vi "Verdi-V5-Main.vi"() -> ()   [LabVIEW 2019]
panel:
  in  "Laser":bool
  out "Power":string
  out "Shutter":bool
  out "Laser":bool
  out "StatusBar":string
  in  "Custom Command":string
  in  "Exit":bool
  in  "Resource":refnum<visa-resource-name>
  out "Response":string
  in  "Query":bool
  in  "Write":bool
  in  "Shutter":bool
  # "Verdi-V5 Control"
  # "W"
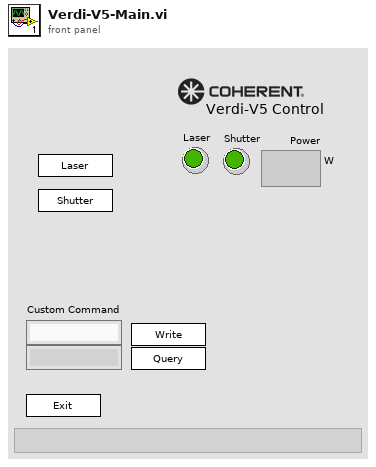
[diagram p1: front panel]
types:
  T1 = enum32{"Invalid", "Standard", "Closed", "Hidden", "Minimized", "Maximized"}
  T2 = enum32{"invalid app kind", "Development System", "Run Time System", "Student Edition", "Embedded LabVIEW", "Evaluation", "Custom"}
  T3 = cluster{"Core":cluster{"Current VI Reference":refnum<vi>, "Close Panel on Exit?":bool}, "Your Boolean data":bool, "Your string data":string, "Resource":refnum<visa-resource-name>}
  T4 = cluster{"Current VI Reference":refnum<vi>, "Close Panel on Exit?":bool}
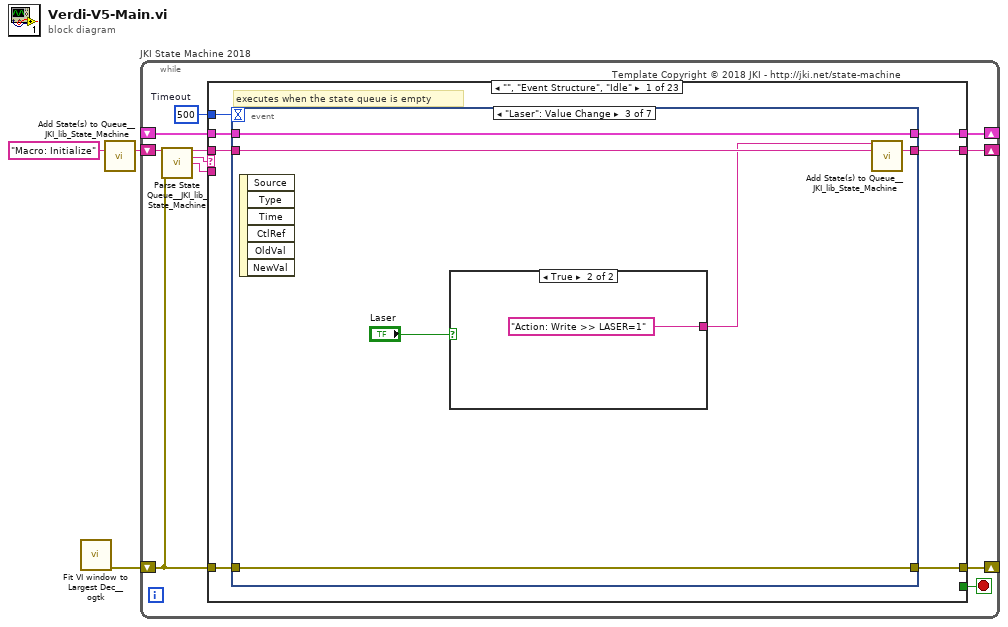
[diagram p0: block diagram]
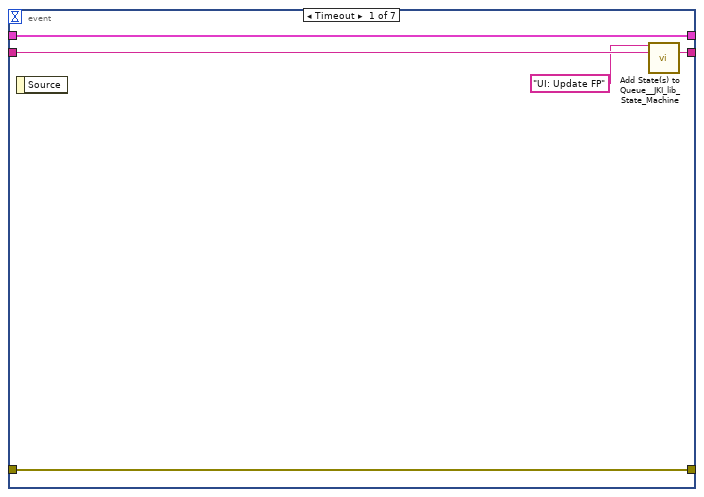
[diagram p2: hidden frame]
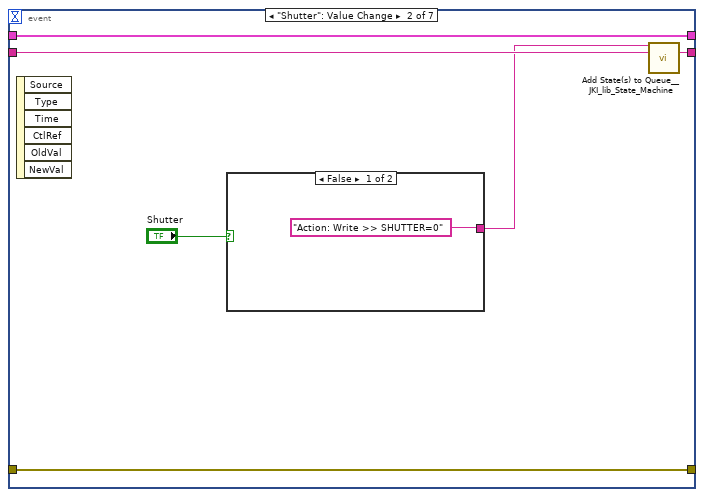
[diagram p3: hidden frame]
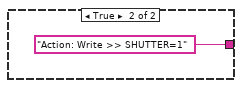
[diagram p4: hidden frame]
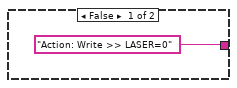
[diagram p5: hidden frame]
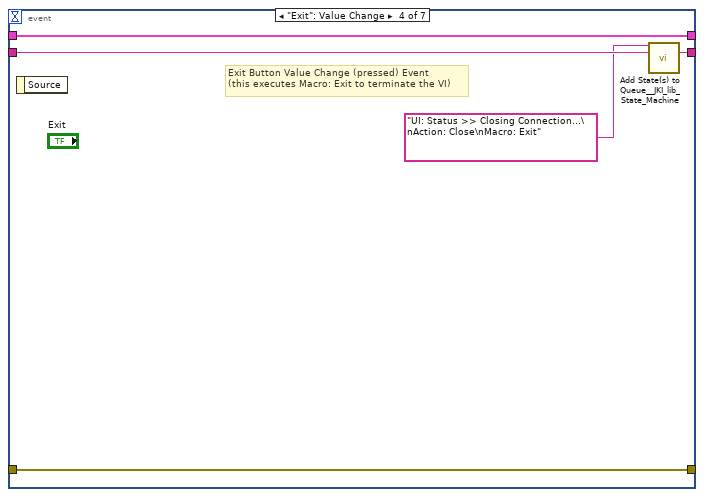
[diagram p6: hidden frame]
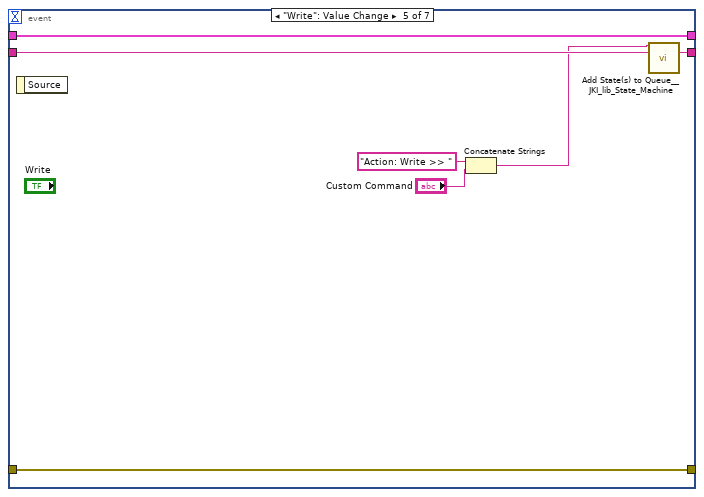
[diagram p7: hidden frame]
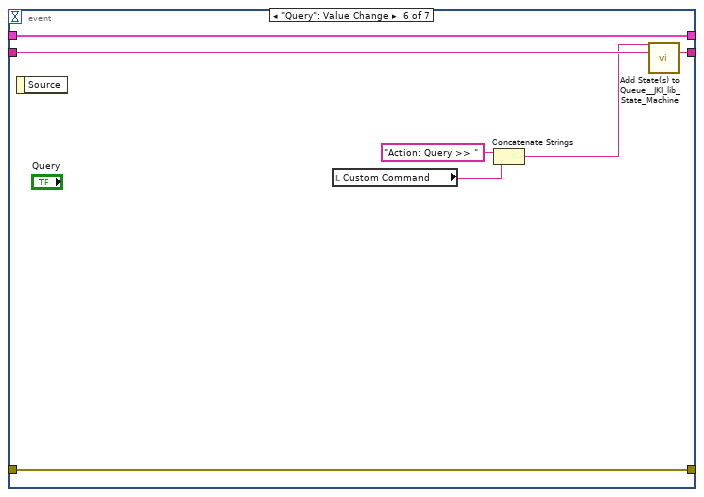
[diagram p8: hidden frame]
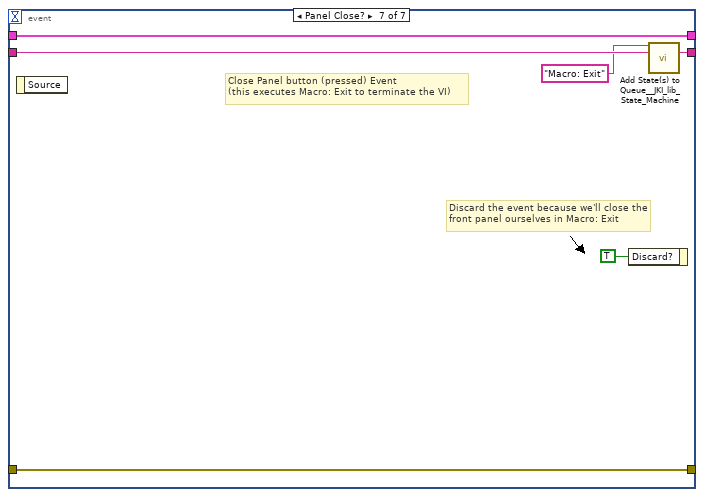
[diagram p9: hidden frame]
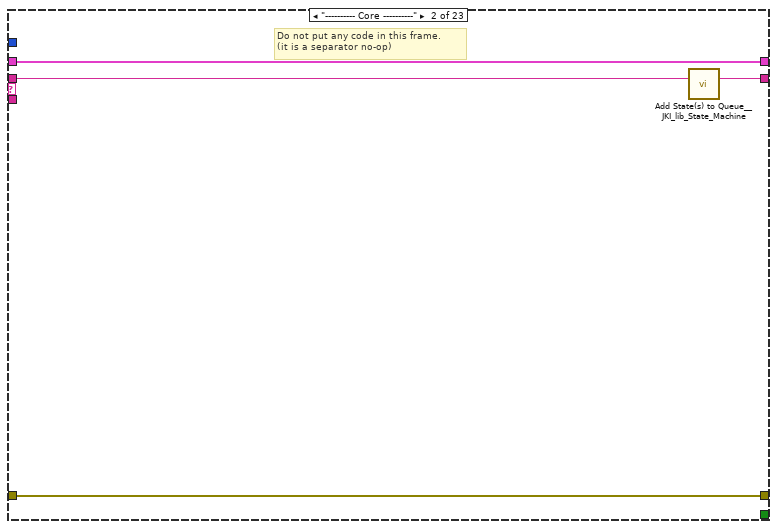
[diagram p10: hidden frame]
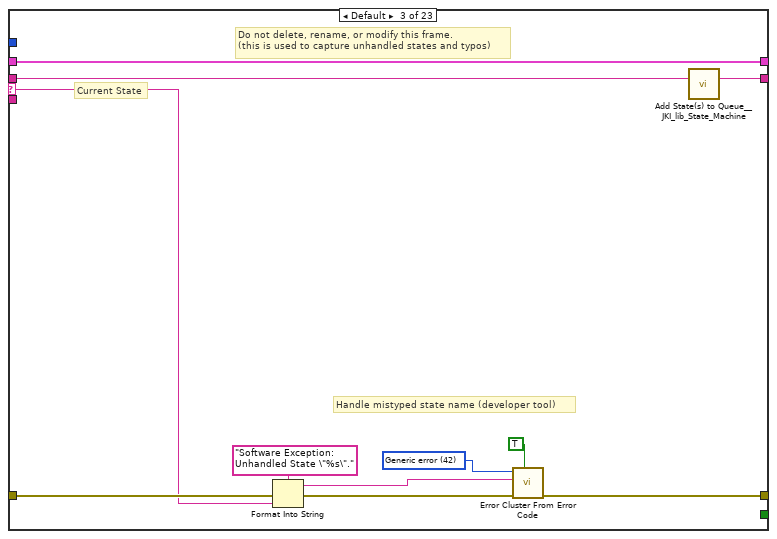
[diagram p11: hidden frame]
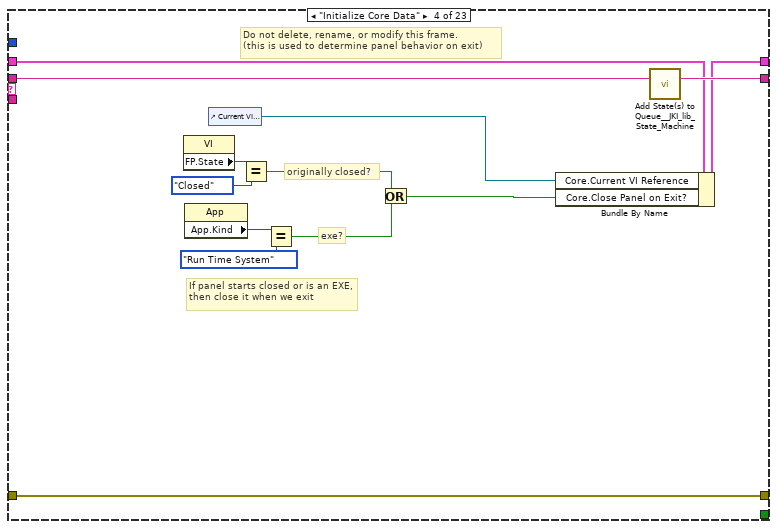
[diagram p12: hidden frame]
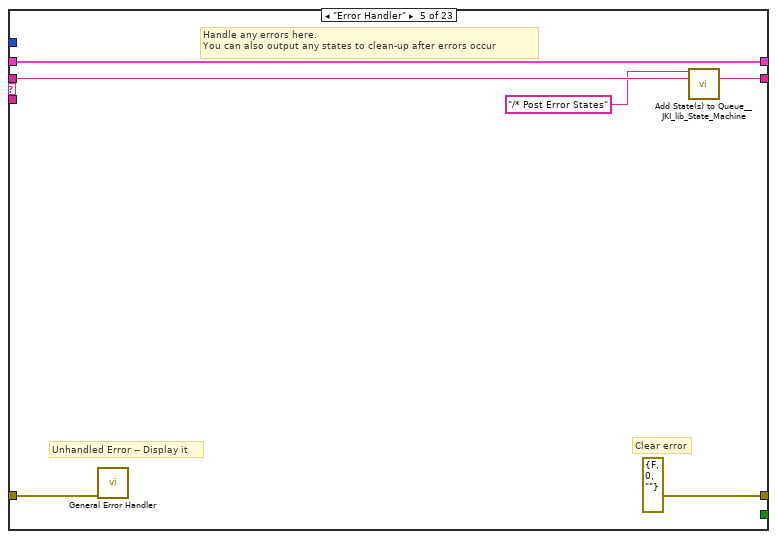
[diagram p13: hidden frame]
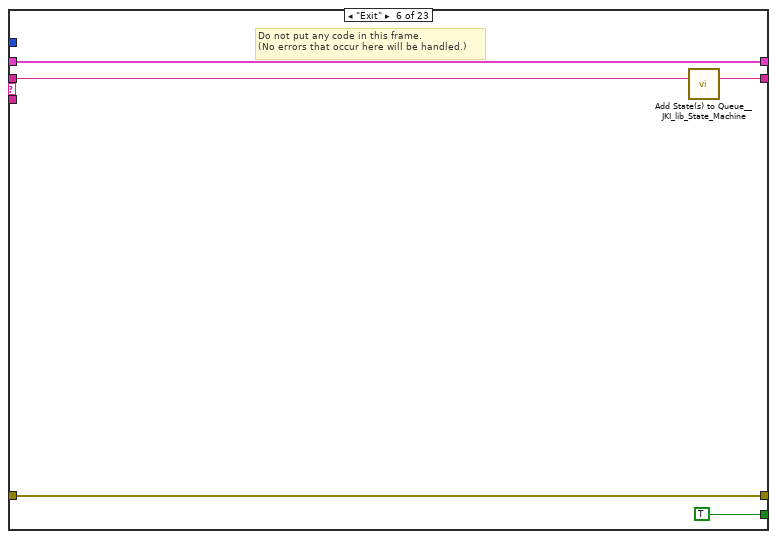
[diagram p14: hidden frame]
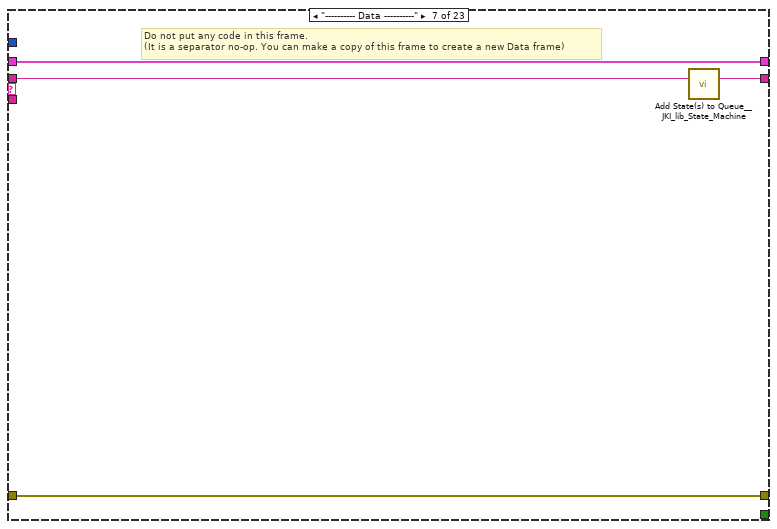
[diagram p15: hidden frame]
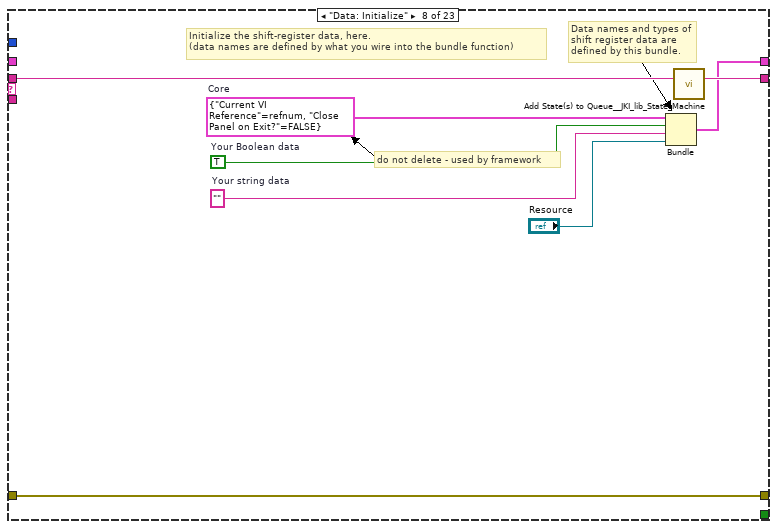
[diagram p16: hidden frame]
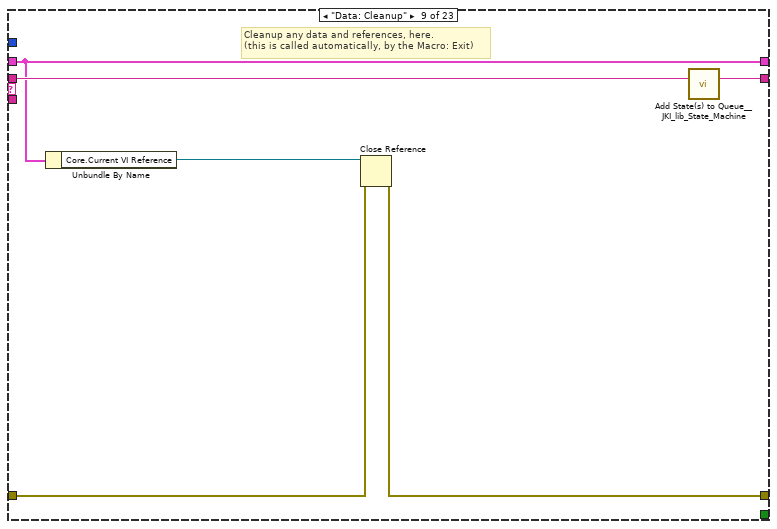
[diagram p17: hidden frame]
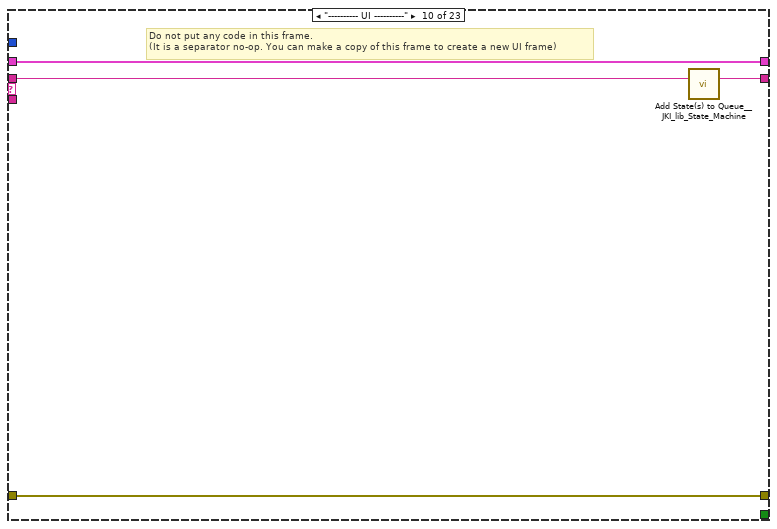
[diagram p18: hidden frame]
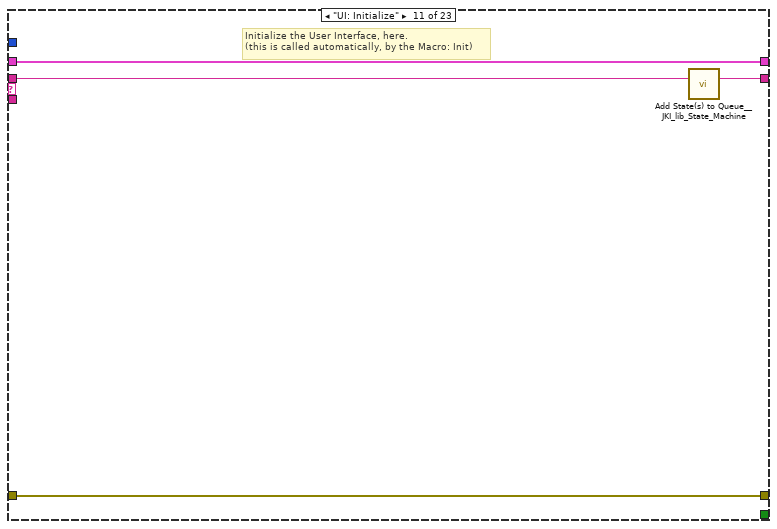
[diagram p19: hidden frame]
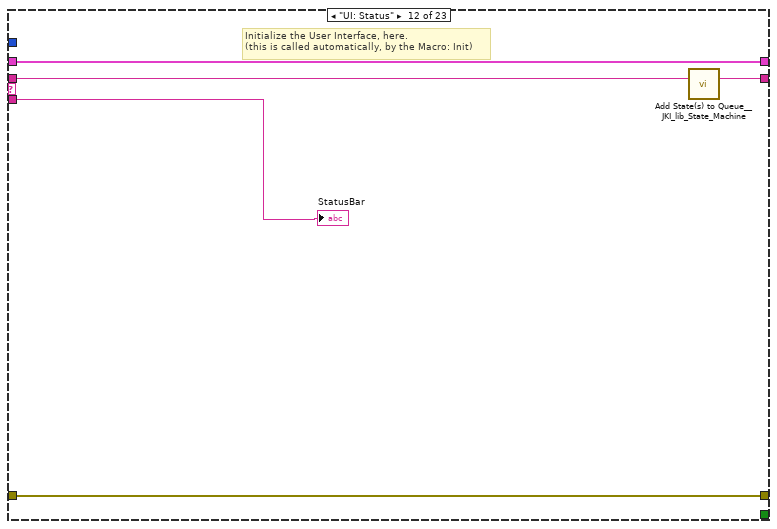
[diagram p20: hidden frame]
diagram:
  n1 = call <userlib>:"Fit VI window to Largest Dec__ogtk.vi"() -> ("error out"=w1:errorcluster)  [unwired: 6 in, 1 out]
  n2 = call <vilib>:"Add State(s) to Queue__JKI_lib_State_Machine.vi"("State(s) in (\"\")"="Macro: Initialize") -> ("States Out"=w3:string)  [unwired: 14 in]
  n3 = while "JKI State Machine 2018" {
    shift-right: [w7] -> _
    shift-left: _ -> [w6]
    shift-right: [w10] -> _
    shift-left: w1 -> [w4]
    shift-right: [w9] -> _
    shift-left: w3 -> [w11]
    stop <- w8 stop-if-true
    w5 = 500  # Timeout
    # "Template Copyright © 2018 JKI - http://jki.net/state-machine"
    n4 = call <vilib>:"Parse State Queue__JKI_lib_State_Machine.vi"("State Queue"=w11, "Error In (no error)"=w4) -> ("Remaining States"=w13:string, "Current State"=w14:string, "Arguments"=w12:string)  [unwired: 11 in]
    n5 = case shown="\"\", \"Event Structure\", \"Idle\"" w14 {
      selector: w14 -> [_ _ w72 _ _ _ _ _ _ _ _ _ _ _ _ _ _ _ _ _ _ _ _]
      tunnel: w13 -> [w21 w71 w76 w95 w101 w106 w110 w118 w124 w128 w132 w137 w159 w165 w176 w245 w250 w260 w264 w274 w280 w289 w299]
      tunnel: w12 -> [_ _ _ _ _ _ _ _ _ _ _ w133 _ w160 w170 _ _ _ _ _ _ w281 w291]
      tunnel: w6 -> [w19 w68 w74 w88 w98 w104 w107 _ w119 w125 w130 w135 w153 w163 w172 w242 w247 w257 w261 w272 w278 w287 w297]
      tunnel: [w18 w69 w78 w92 errorcluster {"status"=FALSE, "code"=0, "source"=""} ("error out") w103 w108 w115 w120 w126 w129 w134 w150 w161 w173 w243 w248 w258 w262 w269 w277 w282 w295] -> w10
      tunnel: w4 -> [w17 w69 w77 w92 w97 w103 w108 w115 w121 w126 w129 w134 w157 w162 w174 w243 w248 w258 w262 w270 w276 w283 w294]
      tunnel: [w20 w70 w75 w94 w100 w105 w109 w117 w123 w127 w131 w136 w158 w164 w175 w244 w249 w259 w263 w273 w279 w288 w298] -> w9
      tunnel: [_ _ _ _ _ TRUE _ _ _ _ _ _ _ _ _ _ _ _ _ _ _ _ _] -> w8
      tunnel: [w16 w68 w74 w93 w98 w104 w107 w116 w119 w125 w130 w135 w152 w163 w172 w242 w247 w257 w261 w271 w278 w286 w296] -> w7
      tunnel: w5 -> [w15 _ _ _ _ _ _ _ _ _ _ _ _ _ _ _ _ _ _ _ _ _ _]
      frame "", "Event Structure", "Idle" {
        # "executes when the state queue is empty"
        n6 = event shown="[2] \"Laser\": Value Change" {
          selector: _ -> [_ _ _ _ _ _ _]
          dyn-events: _ -> [_ _ _ _ _ _ _]
          timeout: w15 -> [_ _ _ _ _ _ _]
          tunnel: w21 -> [w26 w32 w40 w47 w54 w61 w67]
          tunnel: [w25 w31 w39 w46 w53 w60 w66] -> w20
          tunnel: w19 -> [w23 w29 w37 w44 w51 w58 w64]
          tunnel: [w24 w30 w38 w45 w52 w59 w65] -> w18
          tunnel: w17 -> [w24 w30 w38 w45 w52 w59 w65]
          tunnel: [w23 w29 w37 w44 w51 w58 w64] -> w16
          event Timeout {
            n7 = event-data() -> ()  [unwired: 1 in, 1 out]
            n8 = call <vilib>:"Add State(s) to Queue__JKI_lib_State_Machine.vi"("State(s) in Front (\"\")"="UI: Update FP" ("State(s) in Front (\"\")"), "State(s) in (\"\")"=w26) -> ("States Out"=w25:string)  [unwired: 13 in]
          }
          event "Shutter": Value Change {
            n9 = event-data() -> ()  [unwired: 1 in, 6 out]
            n10 = case shown="False" "Shutter" {
              tunnel: ["Action: Write >> SHUTTER=0" "Action: Write >> SHUTTER=1"] -> w28
              frame False {
              }
              frame True {
              }
            }
            n11 = call <vilib>:"Add State(s) to Queue__JKI_lib_State_Machine.vi"("State(s) in Front (\"\")"=w28, "State(s) in (\"\")"=w32) -> ("States Out"=w31:string)  [unwired: 13 in]
          }
          event "Laser": Value Change {
            n12 = event-data() -> ()  [unwired: 1 in, 6 out]
            n13 = case shown="True" "Laser" {
              tunnel: ["Action: Write >> LASER=0" "Action: Write >> LASER=1"] -> w36
              frame False {
              }
              frame True {
              }
            }
            n14 = call <vilib>:"Add State(s) to Queue__JKI_lib_State_Machine.vi"("State(s) in Front (\"\")"=w36, "State(s) in (\"\")"=w40) -> ("States Out"=w39:string)  [unwired: 13 in]
          }
          event "Exit": Value Change {
            # "Exit Button Value Change (pressed) Event\n(this executes Macro: Exit to terminate the VI)"
            n15 = event-data() -> ()  [unwired: 1 in, 1 out]
            n16 = call <vilib>:"Add State(s) to Queue__JKI_lib_State_Machine.vi"("State(s) in Front (\"\")"="UI: Status >> Closing Connection...\nAction: Close\nMacro: Exit", "State(s) in (\"\")"=w47) -> ("States Out"=w46:string)  [unwired: 13 in]
          }
          event "Write": Value Change {
            n17 = event-data() -> ()  [unwired: 1 in, 1 out]
            n18 = Concatenate Strings("Action: Write >> " ("string"), "Custom Command") -> (w49:string)
            n19 = call <vilib>:"Add State(s) to Queue__JKI_lib_State_Machine.vi"("State(s) in Front (\"\")"=w49, "State(s) in (\"\")"=w54) -> ("States Out"=w53:string)  [unwired: 13 in]
          }
          event "Query": Value Change {
            n20 = event-data() -> ()  [unwired: 1 in, 1 out]
            n21 = local read "Custom Command"() -> (w55:string)
            n22 = Concatenate Strings("Action: Query >> " ("string"), w55) -> (w56:string)
            n23 = call <vilib>:"Add State(s) to Queue__JKI_lib_State_Machine.vi"("State(s) in Front (\"\")"=w56, "State(s) in (\"\")"=w61) -> ("States Out"=w60:string)  [unwired: 13 in]
          }
          event Panel Close? {
            # "Discard the event because we'll close the front panel ourselves in Macro: Exit"
            # "Close Panel button (pressed) Event\n(this executes Macro: Exit to terminate the VI)"
            n24 = event-data() -> ()  [unwired: 1 in, 1 out]
            n25 = event-data("Discard?"=TRUE) -> ()  [unwired: 1 in, 1 out]
            n26 = call <vilib>:"Add State(s) to Queue__JKI_lib_State_Machine.vi"("State(s) in Front (\"\")"="Macro: Exit", "State(s) in (\"\")"=w67) -> ("States Out"=w66:string)  [unwired: 13 in]
          }
        }
      }
      frame "---------- Core ----------" {
        # "Do not put any code in this frame.\n(it is a separator no-op)"
        n27 = call <vilib>:"Add State(s) to Queue__JKI_lib_State_Machine.vi"("State(s) in (\"\")"=w71) -> ("States Out"=w70:string)  [unwired: 14 in]
      }
      frame Default {
        w81 = 42 items=["No error", "Argument error", "Memory is full", "Out of zone", "End of file", "File already open", "Generic file I/O error", "File not found", "File permission error", "Disk is full", "Duplicate path", "Too many files open", "System feature not enabled", "Resource file not found", "Cannot add resource", "Resource not found", "Image not found", "Image memory error", "Pen does not exist", "Config type invalid", "Config token not found", "Config parse error", "Config memory error", "Bad external code format", "Bad external code offset", "External code not present", "Null window", "Destroy window error", "Null menu", "Print aborted", "Bad print record", "Print driver error", "Windows error during printing", "Memory error during printing", "Print dialog error", "Generic print error", "Invalid device refnum", "Device not found", "Device parameter error", "Device unit error", "Cannot open device", "Device call aborted", "Generic error", "Cancelled by user", "Object ID too low", "Object ID too high", "Object not in heap", "Unknown heap", "Unknown object (invalid DefProc)", "Unknown object (DefProc not in table)", "Message out of range", "Invalid (null) method", "Unknown message", "Manager call not supported", "Bad address", "Network operation in progress", "Network operation timed out", "Connection is busy", "Network attribute not supported", "Network error", "Address in use", "System out of memory", "Connection aborted", "Connection refused", "Not connected", "Already connected", "Connection closed", "Initialization error (interapplication manager)", "Bad occurrence", "Wait on unbound occurrence handler", "Occurrence queue overflow", "Datalog type conflict", "Unused", "Unrecognized type (interapplication manager)", "Memory corrupt", "Failed to make temporary DLL", "Old CIN version", "Drag socket not found", "Failed to load drop-object", "Failed to register OLE object", "Failed to release OLE object", "Format specifier type mismatch", "Unknown format specifier", "Too few format specifiers", "Too many format specifiers", "Scan failed", "Newer CIN version", "Error converting to variant", "Runtime menu error", "Password tampered", "Variant attribute not found", "Incompatible variant data type", "Event data is not available", "Event Store is not present", "Occurrence is not found", "Event Queue is not created", "Event info is not available", "Refnum passed is NULL", "Error retrieving Class GUID", "Error retrieving CoClass GUID", "Error retrieving TypeLib GUID.", "Bad built application magic bytes.", "Specific driver is different from the specific driver associated with the Logical Name.", "There is no session opened to the class driver.", "Max Error", "MAX - Error with config objects", "MAX - Error loading configuration", "MAX - Group not supported"]
        # "Current State"
        # "Do not delete, rename, or modify this frame.\n(this is used to capture unhandled states and typos)"
        # "Handle mistyped state name (developer tool)"
        n28 = Format Into String(format string="Software Exception: Unhandled State \"%s\"." ("message"), error in=w77, w72) -> (resulting string=w80:string, error out=w79:errorcluster)  [unwired: 1 in]
        n29 = call <vilib>:"Error Cluster From Error Code.vi"("show call chain? (False)"=TRUE, "error in (no error)"=w79, "error message (\"\")"=w80, "error code (0)"=w81) -> ("error out"=w78:errorcluster)  [unwired: 5 in]
        n30 = call <vilib>:"Add State(s) to Queue__JKI_lib_State_Machine.vi"("State(s) in (\"\")"=w76) -> ("States Out"=w75:string)  [unwired: 14 in]
      }
      frame "Initialize Core Data" {
        # "Do not delete, rename, or modify this frame.\n(this is used to determine panel behavior on exit)"
        # "originally closed?"
        # "exe?"
        # "If panel starts closed or is an EXE, then close it when we exit"
        n31 = property class="VI"() -> ("FP.State"=w85:T1)  [unwired: 2 in, 2 out]
        n32 = property class="App"() -> ("App.Kind"=w91:T2)  [unwired: 2 in, 2 out]
        n33 = control-ref of="Current VI Reference"() -> (w86:refnum<vi>)
        n34 = Equal?(x=w85, y=T1."Closed" ("Front Panel Window:State")) -> (x = y?=w83:bool)
        n35 = Equal?(x=w91, y=T2."Run Time System" ("Application:Kind")) -> (x = y?=w89:bool)
        n36 = Or(x=w83, y=w89) -> (x .or. y?=w87:bool)
        n37 = Bundle By Name(cluster=w88, "Core.Current VI Reference"=w86, "Core.Close Panel on Exit?"=w87) -> (w93:T3)
        n38 = call <vilib>:"Add State(s) to Queue__JKI_lib_State_Machine.vi"("State(s) in (\"\")"=w95) -> ("States Out"=w94:string)  [unwired: 14 in]
      }
      frame "Error Handler" {
        # "Unhandled Error -- Display it"
        # "Handle any errors here.\nYou can also output any states to clean-up after errors occur"
        # "Clear error"
        n39 = call <vilib>:"General Error Handler.vi"("error in (no error)"=w97) -> ()  [unwired: 10 in, 5 out]
        n40 = call <vilib>:"Add State(s) to Queue__JKI_lib_State_Machine.vi"("State(s) in Front (\"\")"="/* Post Error States", "State(s) in (\"\")"=w101) -> ("States Out"=w100:string)  [unwired: 13 in]
      }
      frame "Exit" {
        # "Do not put any code in this frame.\n(No errors that occur here will be handled.)"
        n41 = call <vilib>:"Add State(s) to Queue__JKI_lib_State_Machine.vi"("State(s) in (\"\")"=w106) -> ("States Out"=w105:string)  [unwired: 14 in]
      }
      frame "---------- Data ----------" {
        # "Do not put any code in this frame.\n(It is a separator no-op. You can make a copy of this frame to create a new Data frame)"
        n42 = call <vilib>:"Add State(s) to Queue__JKI_lib_State_Machine.vi"("State(s) in (\"\")"=w110) -> ("States Out"=w109:string)  [unwired: 14 in]
      }
      frame "Data: Initialize" {
        w112 = T4 {"Current VI Reference"=refnum, "Close Panel on Exit?"=FALSE}  # Core
        w114 = TRUE  # Your Boolean data
        w113 = ""  # Your string data
        # "do not delete - used by framework"
        # "Data names and types of shift register data are defined by this bundle."
        # "Initialize the shift-register data, here.\n(data names are defined by what you wire into the bundle function)"
        n43 = Bundle("Core"=w112, "Your Boolean data"=w114, "Your string data"=w113, "Resource"="Resource") -> (w116:T3)  [unwired: 1 in]
        n44 = call <vilib>:"Add State(s) to Queue__JKI_lib_State_Machine.vi"("State(s) in (\"\")"=w118) -> ("States Out"=w117:string)  [unwired: 14 in]
      }
      frame "Data: Cleanup" {
        # "Cleanup any data and references, here.\n(this is called automatically, by the Macro: Exit)"
        n45 = Unbundle By Name(w119) -> ("Core.Current VI Reference"=w122:refnum<vi>)
        n46 = Close Reference(reference=w122, error in (no error)=w121) -> (error out=w120:errorcluster)
        n47 = call <vilib>:"Add State(s) to Queue__JKI_lib_State_Machine.vi"("State(s) in (\"\")"=w124) -> ("States Out"=w123:string)  [unwired: 14 in]
      }
      frame "---------- UI ----------" {
        # "Do not put any code in this frame.\n(It is a separator no-op. You can make a copy of this frame to create a new UI frame)"
        n48 = call <vilib>:"Add State(s) to Queue__JKI_lib_State_Machine.vi"("State(s) in (\"\")"=w128) -> ("States Out"=w127:string)  [unwired: 14 in]
      }
      frame "UI: Initialize" {
        # "Initialize the User Interface, here.\n(this is called automatically, by the Macro: Init)"
        n49 = call <vilib>:"Add State(s) to Queue__JKI_lib_State_Machine.vi"("State(s) in (\"\")"=w132) -> ("States Out"=w131:string)  [unwired: 14 in]
      }
      frame "UI: Status" {
        # "Initialize the User Interface, here.\n(this is called automatically, by the Macro: Init)"
        n50 = call <vilib>:"Add State(s) to Queue__JKI_lib_State_Machine.vi"("State(s) in (\"\")"=w137) -> ("States Out"=w136:string)  [unwired: 14 in]
        "StatusBar" <- w133
      }
      frame "UI: Update FP" {
        # "Initialize the User Interface, here.\n(this is called automatically, by the Macro: Init)"
        n51 = Unbundle By Name(w153) -> ("Resource"=w156:refnum<visa-resource-name>)
        n52 = call "Query.vi"("error in (no error)"=w157, "Command"="?L", "VISA resource name"=w156) -> ("error out"=w149:errorcluster, "Response"=w145:string, "VISA resource name out"=w155:refnum<visa-resource-name>)  [unwired: 5 in, 1 out]
        n53 = Decimal String To Number(string=w145) -> (number=w143:i32)  [unwired: 2 in, 1 out]
        n54 = Greater Than 0?(x=w143) -> (x > 0?=→"Laser":bool)
        n55 = call "Query.vi"("error in (no error)"=w149, "Command"="?S", "VISA resource name"=w155) -> ("error out"=w148:errorcluster, "Response"=w146:string, "VISA resource name out"=w154:refnum<visa-resource-name>)  [unwired: 5 in, 1 out]
        n56 = Decimal String To Number(string=w146) -> (number=w142:i32)  [unwired: 2 in, 1 out]
        n57 = Greater Than 0?(x=w142) -> (x > 0?=→"Shutter":bool)
        n58 = call "Query.vi"("error in (no error)"=w148, "Command"="?LIGHT", "VISA resource name"=w154) -> ("error out"=w150:errorcluster, "Response"=→"Power":string, "VISA resource name out"=w151:refnum<visa-resource-name>)  [unwired: 5 in, 1 out]
        n59 = Bundle By Name(cluster=w153, "Resource"=w151) -> (w152:T3)
        n60 = call <vilib>:"Add State(s) to Queue__JKI_lib_State_Machine.vi"("State(s) in (\"\")"=w159) -> ("States Out"=w158:string)  [unwired: 14 in]
      }
      frame "UI: Cursor Set" {
        # "Argument"
        # "Set and Unset Cursor Busy.\n(Usage: \"UI: Cursor Set >> Busy|Idle\")"
        n61 = case shown="\"Idle\", Default" w160 {
          tunnel: w162 -> [w167 w169]
          tunnel: [w166 w168] -> w161
          frame "Idle", Default {
            n62 = call <vilib>:"Unset Busy.vi"("error in (no error)"=w167) -> ("error out"=w166:errorcluster)  [unwired: 10 in]
          }
          frame "Busy" {
            n63 = call <vilib>:"Set Busy.vi"("error in (no error)"=w169) -> ("error out"=w168:errorcluster)  [unwired: 9 in, 1 out]
          }
        }
        n64 = call <vilib>:"Add State(s) to Queue__JKI_lib_State_Machine.vi"("State(s) in (\"\")"=w165) -> ("States Out"=w164:string)  [unwired: 14 in]
      }
      frame "UI: Front Panel State" {
        # "Argument"
        # "Set Front Panel Open or Closed\n(Usage: \"UI: Front Panel State >> Open|Close\")"
        n65 = Unbundle By Name(w172) -> ("Core.Current VI Reference"=w171:refnum<vi>)
        n66 = case shown="\"Minimize\", \"Minimized\"" w170 {
          tunnel: w174 -> [w182 w197 w208 w221 w234]
          tunnel: [w184 w198 w210 w223 w236] -> w173
          tunnel: w171 -> [w183 w195 w209 w222 w235]
          frame "Open", "Standard", Default {
            w177 = T1."Standard" ("State")
            n67 = property class="VI"(reference=w183, error in=w182) -> (reference out=w180:refnum<vi>, error out=w181:errorcluster, "FP.State"=w179:T1)
            n68 = Not Equal?(x=w179, y=w177) -> (x != y?=w178:bool)
            n69 = case shown="True" w178 {
              tunnel: [w188 w190] -> w184
              tunnel: w181 -> [w187 w190]
              tunnel: w180 -> [w186 _]
              tunnel: w177 -> [w185 _]
              frame True {
                n70 = invoke class="VI" method="FP.Open"(reference=w186, error in=w187, "Activate"=TRUE, "State"=w185) -> (error out=w188:errorcluster)  [unwired: 1 in, 4 out]
              }
              frame False {
              }
            }
          }
          frame "Close", "Closed" {
            n71 = property class="VI"(reference=w195, error in=w197) -> (reference out=w194:refnum<vi>, error out=w196:errorcluster, "FP.State"=w192:T1)
            n72 = Not Equal?(x=w192, y=T1."Closed" ("Front Panel Window:State")) -> (x != y?=w191:bool)
            n73 = case shown="True" w191 {
              tunnel: [w199 w202] -> w198
              tunnel: w196 -> [w199 w201]
              tunnel: w194 -> [_ w200]
              frame False {
              }
              frame True {
                n74 = invoke class="VI" method="FP.Close"(reference=w200, error in=w201) -> (error out=w202:errorcluster)  [unwired: 1 in, 2 out]
              }
            }
          }
          frame "Hidden", "Hide" {
            w203 = T1."Hidden" ("State")
            n75 = property class="VI"(reference=w209, error in=w208) -> (reference out=w206:refnum<vi>, error out=w207:errorcluster, "FP.State"=w205:T1)
            n76 = Not Equal?(x=w205, y=w203) -> (x != y?=w204:bool)
            n77 = case shown="True" w204 {
              tunnel: [w214 w215] -> w210
              tunnel: w207 -> [w213 w215]
              tunnel: w206 -> [w212 _]
              tunnel: w203 -> [w211 _]
              frame True {
                n78 = invoke class="VI" method="FP.Open"(reference=w212, error in=w213, "State"=w211) -> (error out=w214:errorcluster)  [unwired: 2 in, 4 out]
              }
              frame False {
              }
            }
          }
          frame "Minimize", "Minimized" {
            w216 = T1."Minimized" ("State")
            n79 = property class="VI"(reference=w222, error in=w221) -> (reference out=w219:refnum<vi>, error out=w220:errorcluster, "FP.State"=w218:T1)
            n80 = Not Equal?(x=w218, y=w216) -> (x != y?=w217:bool)
            n81 = case shown="True" w217 {
              tunnel: [w227 w228] -> w223
              tunnel: w220 -> [w226 w228]
              tunnel: w219 -> [w225 _]
              tunnel: w216 -> [w224 _]
              frame True {
                n82 = invoke class="VI" method="FP.Open"(reference=w225, error in=w226, "State"=w224) -> (error out=w227:errorcluster)  [unwired: 2 in, 4 out]
              }
              frame False {
              }
            }
          }
          frame "Maximize", "Maximized" {
            w229 = T1."Maximized" ("State")
            n83 = property class="VI"(reference=w235, error in=w234) -> (reference out=w232:refnum<vi>, error out=w233:errorcluster, "FP.State"=w231:T1)
            n84 = Not Equal?(x=w231, y=w229) -> (x != y?=w230:bool)
            n85 = case shown="True" w230 {
              tunnel: [w240 w241] -> w236
              tunnel: w233 -> [w239 w241]
              tunnel: w232 -> [w238 _]
              tunnel: w229 -> [w237 _]
              frame True {
                n86 = invoke class="VI" method="FP.Open"(reference=w238, error in=w239, "State"=w237) -> (error out=w240:errorcluster)  [unwired: 2 in, 4 out]
              }
              frame False {
              }
            }
          }
        }
        n87 = call <vilib>:"Add State(s) to Queue__JKI_lib_State_Machine.vi"("State(s) in (\"\")"=w176) -> ("States Out"=w175:string)  [unwired: 14 in]
      }
      frame "---------- Macro ----------" {
        # "Do not put any code in this frame.\n(It is a separator no-op. You can make a copy of this frame to create a new Macro frame)"
        n88 = call <vilib>:"Add State(s) to Queue__JKI_lib_State_Machine.vi"("State(s) in (\"\")"=w245) -> ("States Out"=w244:string)  [unwired: 14 in]
      }
      frame "Macro: Initialize" {
        w246 = "UI: Status >> Initializing...\nData: Initialize\nInitialize Core Data\nUI: Initialize\nUI: Front Panel State >> Open\nAction: Open"  # UI: Status >> Initializing... Data: Initialize Initialize Core Data UI: Initialize UI: Front Panel State >> Open Action: Open
        # "Initialization Macro\n(This is called once, when the VI starts)"
        n89 = call <vilib>:"Add State(s) to Queue__JKI_lib_State_Machine.vi"("State(s) in Front (\"\")"=w246, "State(s) in (\"\")"=w250) -> ("States Out"=w249:string)  [unwired: 13 in]
      }
      frame "Macro: Exit" {
        # "Exit Macro\n(This is called once, when the VI exits)"
        n90 = Unbundle By Name(w257) -> ("Core.Close Panel on Exit?"=w256:bool)
        n91 = Select(t="UI: Front Panel State >> Close", s=w256, f="") -> (s? t:f=w253:string)
        n92 = call <vilib>:"Add State(s) to Queue__JKI_lib_State_Machine.vi"("State(s) in (\"\")"=w253, "State(s) at Back (\"\")"="Data: Cleanup\nExit") -> ("States Out"=w251:string)  [unwired: 13 in]
        n93 = call <vilib>:"Add State(s) to Queue__JKI_lib_State_Machine.vi"("State(s) in Front (\"\")"=w251, "State(s) in (\"\")"=w260) -> ("States Out"=w259:string)  [unwired: 13 in]
      }
      frame "---------- Action ----------" {
        # "Template Separator\n(You can make a copy of, or modify, this frame)"
        n94 = call <vilib>:"Add State(s) to Queue__JKI_lib_State_Machine.vi"("State(s) in (\"\")"=w264) -> ("States Out"=w263:string)  [unwired: 14 in]
      }
      frame "Action: Open" {
        n95 = call "Open.vi"("error in (no error)"=w270) -> ("error out"=w269:errorcluster, "VISA resource name out"=w268:refnum<visa-resource-name>)  [unwired: 9 in]
        n96 = Bundle By Name(cluster=w272, "Resource"=w268) -> (w271:T3)
        n97 = property class="Instr"(reference=w268) -> ("Intf Inst Name"=w267:string)  [unwired: 1 in, 2 out]
        n98 = Format Into String(format string="UI: Status >> Connected to Verdi on %s " ("initial string"), w267) -> (resulting string=w266:string)  [unwired: 2 in, 1 out]
        n99 = call <vilib>:"Add State(s) to Queue__JKI_lib_State_Machine.vi"("State(s) in Front (\"\")"=w266, "State(s) in (\"\")"=w274) -> ("States Out"=w273:string)  [unwired: 13 in]
      }
      frame "Action: Close" {
        n100 = Unbundle By Name(w278) -> ("Resource"=w275:refnum<visa-resource-name>)
        n101 = call "Close.vi"("error in (no error)"=w276, "VISA resource name"=w275) -> ("error out"=w277:errorcluster)  [unwired: 9 in]
        n102 = call <vilib>:"Add State(s) to Queue__JKI_lib_State_Machine.vi"("State(s) in (\"\")"=w280) -> ("States Out"=w279:string)  [unwired: 14 in]
      }
      frame "Action: Write" {
        n103 = Unbundle By Name(w287) -> ("Resource"=w284:refnum<visa-resource-name>)
        n104 = call "SendCommand.vi"("error in (no error)"=w283, "Command"=w281, "VISA resource name"=w284) -> ("error out"=w282:errorcluster, "VISA resource name out"=w285:refnum<visa-resource-name>)  [unwired: 7 in]
        n105 = Bundle By Name(cluster=w287, "Resource"=w285) -> (w286:T3)
        n106 = call <vilib>:"Add State(s) to Queue__JKI_lib_State_Machine.vi"("State(s) in (\"\")"=w289) -> ("States Out"=w288:string)  [unwired: 14 in]
      }
      frame "Action: Query" {
        # "Template Separator\n(You can make a copy of, or modify, this frame)"
        n107 = Unbundle By Name(w297) -> ("Resource"=w293:refnum<visa-resource-name>)
        n108 = call "Query.vi"("error in (no error)"=w294, "Command"=w291, "VISA resource name"=w293) -> ("error out"=w295:errorcluster, "Response"=→"Response":string, "VISA resource name out"=w292:refnum<visa-resource-name>)  [unwired: 5 in, 1 out]
        n109 = Bundle By Name(cluster=w297, "Resource"=w292) -> (w296:T3)
        n110 = call <vilib>:"Add State(s) to Queue__JKI_lib_State_Machine.vi"("State(s) in (\"\")"=w299) -> ("States Out"=w298:string)  [unwired: 14 in]
      }
    }
  }
